vi "Execute.vi"(8 "error in (no error)":errorcluster, 9 "System in":refnum<class "System.lvclass">, 10 "Command in":refnum<class "Command.lvclass">, 11 "CT-GrabberInWay-State in":refnum<class "CT-GrabberInWay-State.lvclass">) -> (0 "error out":errorcluster, 2 "Next State":refnum<class "State.lvclass">, 3 "CT-GrabberInWay-State out":refnum<class "CT-GrabberInWay-State.lvclass">)   [LabVIEW 2013, in "CT-GrabberInWay-State.lvclass"]
uses:
  CT-GrabberInWay-State.lvclass
  Commands/Command/Command.lvclass
  Systems/System/System.lvclass
  State/State.lvclass
  CT-Energized-State/CT-Energized-State.lvclass
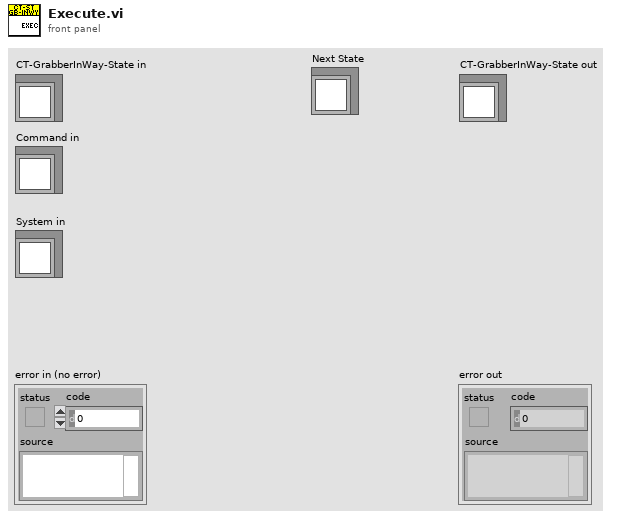
[diagram p1: front panel]
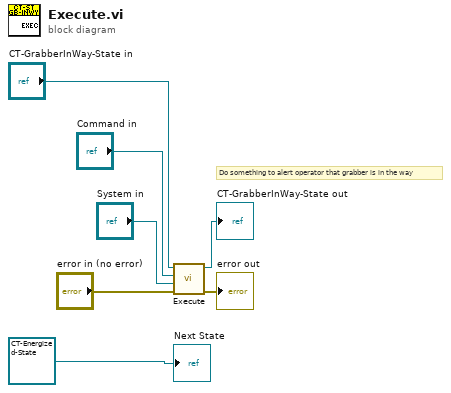
[diagram p0: block diagram]
diagram:
  # "Do something to alert operator that grabber is in the way"
  n1 = call-parent "Execute.vi"("error in (no error)"="error in (no error)", "System in"="System in", "Command in"="Command in", "State in"="CT-GrabberInWay-State in") -> ("error out"=→"error out":errorcluster, "State out"=→"CT-GrabberInWay-State out":refnum<class "CT-GrabberInWay-State.lvclass">)  [unwired: 5 in, 1 out]
  "Next State" <- refnum<class "CT-Energized-State.lvclass"> refnum ("CT-Energized-State.lvclass")
